vi "FTW-TestExecutive-Results-Deserialize.vi"(0 "Serialized Results":string, 11 "error in (no error)":errorcluster) -> (4 "Results":T1 {"Start Time" format="%<%Y-%m-%d %H:%M:%S%03u>T"; "Elapsed Time" format="%<%H:%M:%S%3u>t"}, 15 "error out":errorcluster)   [LabVIEW 2015]
doc: "This VI is intended to be used <b>only by test steps</b> to report their results to the Test Executive"
uses:
  FTW-TestExecutive-Results.ctl
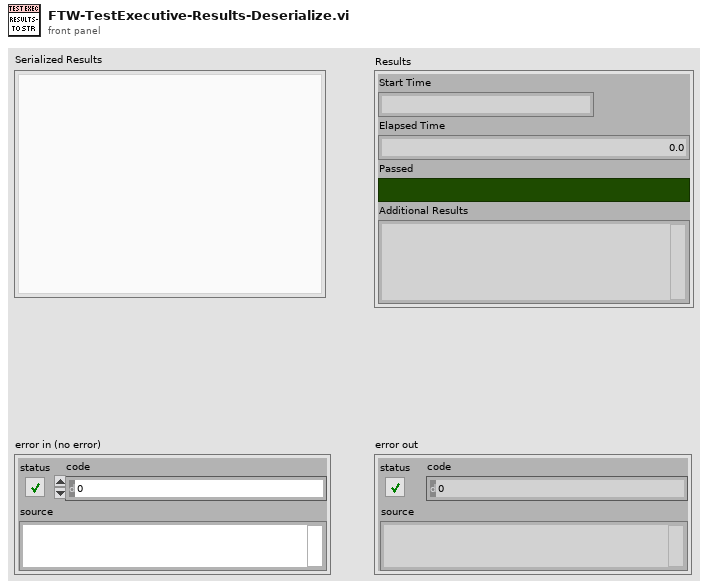
[diagram p1: front panel]
types:
  T1 = typedef "FTW-TestExecutive-Results.ctl" = cluster{"Start Time":timestamp, "Elapsed Time":dbl, "Passed":bool, "Additional Results":string}
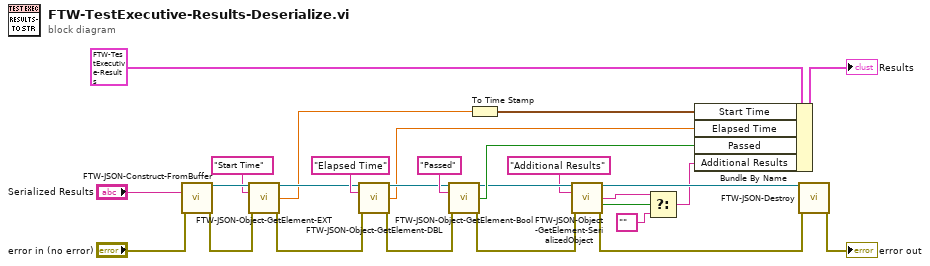
[diagram p0: block diagram]
diagram:
  n1 = call "FTW-JSON-Construct-FromBuffer.vi"("JSON String (UTF-8)"="Serialized Results", "error in"="error in (no error)") -> ("JSON"=w14:refnum<class "FTW-Container.lvclass">, "error out"=w25:errorcluster)  [unwired: 12 in]
  n2 = call "FTW-JSON-Object-GetElement-EXT.vi"("JSON"=w14, "Key"="Start Time", "error in"=w25) -> ("JSON out"=w13:refnum<class "FTW-Container.lvclass">, "Value"=w6:ext, "error out"=w5:errorcluster)  [unwired: 9 in, 1 out]
  n3 = call "FTW-JSON-Object-GetElement-DBL.vi"("JSON"=w13, "Key"="Elapsed Time", "error in"=w5) -> ("JSON out"=w17:refnum<class "FTW-Container.lvclass">, "Value"=w15:dbl, "error out"=w18:errorcluster)  [unwired: 9 in, 1 out]
  n4 = call "FTW-JSON-Object-GetElement-Bool.vi"("JSON"=w17, "Key"="Passed", "error in"=w18) -> ("JSON out"=w10:refnum<class "FTW-Container.lvclass">, "Value"=w19:bool, "error out"=w21:errorcluster)  [unwired: 9 in, 1 out]
  n5 = To Time Stamp(1:w6) -> (0:w11:timestamp)
  n6 = call "FTW-JSON-Object-GetElement-SerializedObject.vi"("JSON"=w10, "Key"="Additional Results", "error in"=w21) -> ("JSON out"=w9:refnum<class "FTW-Container.lvclass">, "Value"=w3:string, "Found"=w4:bool, "error out"=w7:errorcluster)  [unwired: 8 in, 1 out]
  n7 = Select(t=w3, s=w4, f="" ("empty string")) -> (s? t:f=w1:string)
  n8 = Bundle By Name(cluster=T1 {"Start Time"=timestamp(0 s since 1904-01-01), "Elapsed Time"=0.0, "Passed"=FALSE, "Additional Results"=""} ("Results"), "Start Time"=w11, "Elapsed Time"=w15, "Passed"=w19, "Additional Results"=w1) -> (→"Results":T1)
  n9 = call "FTW-JSON-Destroy.vi"("JSON"=w9, "error in"=w7) -> ("error out"=→"error out":errorcluster)  [unwired: 13 in]
